vi "Pre Launch Init.vi"(11 "Base Software_Tools in":refnum<class "Main.lvclass">) -> (0 "error out":errorcluster, 3 "Base Software_Tools out":refnum<class "Main.lvclass">)   [LabVIEW 2023, in "Main.lvlib" / "Main.lvclass"]
uses:
  Project/Main.lvclass
  builds/Engine/Engine.lvlibp/Project/Engine.lvclass
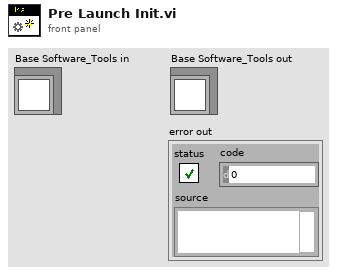
[diagram p1: front panel]
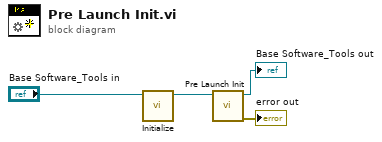
[diagram p0: block diagram]
diagram:
  n1 = call "Initialize.vi"("Base Software in"="Base Software_Tools in") -> ("Base Software out"=w2:refnum<class "Main.lvclass">)  [unwired: 9 in, 1 out]
  n2 = call-parent "Pre Launch Init.vi"("Engine_Tools in"=w2) -> ("error out"=→"error out":errorcluster, "Engine_Tools out"=→"Base Software_Tools out":refnum<class "Main.lvclass">)  [unwired: 9 in]
